vi "SimpleJsonQuery.vi"(8 "error in":errorcluster, 10 "Lookup":string, 11 "String":string) -> (0 "error out":errorcluster, 2 "Value As Numeric":dbl, 3 "Value As String":string)   [LabVIEW 2020]
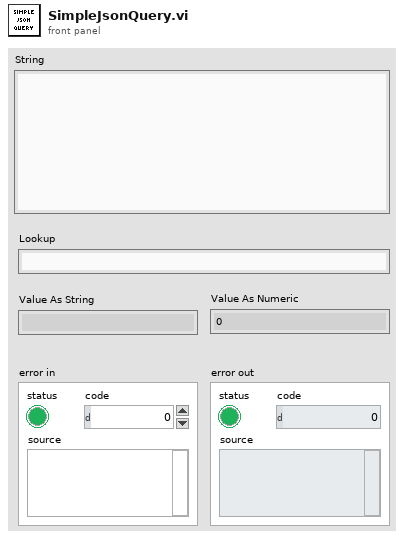
[diagram p1: front panel]
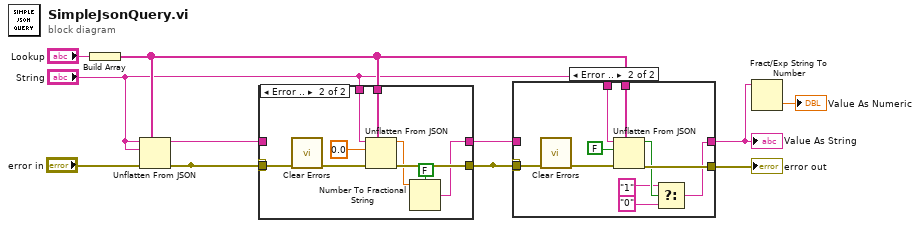
[diagram p0: block diagram]
diagram:
  n1 = Build Array("Lookup") -> (w10:string[])
  n2 = Unflatten From JSON(path=w10, JSON string="String", type and defaults="String", error in (no error)="error in") -> (value=w5:string, error out=w6:errorcluster)  [unwired: 3 in]
  n3 = case shown="Error .." w6 {
    selector: w6 -> [_ w16]
    tunnel: w10 -> [_ w22]
    tunnel: "String" -> [_ w21]
    tunnel: w6 -> [w13 _]
    tunnel: [w13 w19] -> w4
    tunnel: w5 -> [w12 _]
    tunnel: [w12 w17] -> w3
    frame No Error {
    }
    frame Error {
      n4 = call <vilib>:"Clear Errors.vi"("error in (no error)"=w16) -> ("error out"=w15:errorcluster)  [unwired: 5 in, 1 out]
      n5 = Unflatten From JSON(path=w22, JSON string=w21, type and defaults=0.0, error in (no error)=w15) -> (value=w18:dbl, error out=w19:errorcluster)  [unwired: 3 in]
      n6 = Number To Fractional String(use system decimal point (T)=FALSE, number=w18) -> (F-format string=w17:string)  [unwired: 2 in]
    }
  }
  n7 = case shown="Error .." w4 {
    tunnel: w10 -> [_ w34]
    tunnel: "String" -> [_ w33]
    tunnel: w4 -> [w24 w26]
    tunnel: [w24 w31] -> w7
    tunnel: [w23 w27] -> w2
    tunnel: w3 -> [w23 _]
    frame No Error {
    }
    frame Error {
      n8 = call <vilib>:"Clear Errors.vi"("error in (no error)"=w26) -> ("error out"=w25:errorcluster)  [unwired: 5 in, 1 out]
      n9 = Unflatten From JSON(path=w34, JSON string=w33, type and defaults=FALSE, error in (no error)=w25) -> (value=w30:bool, error out=w31:errorcluster)  [unwired: 3 in]
      n10 = Select(t="1", s=w30, f="0") -> (s? t:f=w27:string)
    }
  }
  "Value As String" <- w2
  "error out" <- w7
  n11 = Fract/Exp String To Number(string=w2) -> (number=→"Value As Numeric":dbl)  [unwired: 3 in, 1 out]
